vi "Parent.vi"(10 "Label.Text":string, 11 "Parent in":string) -> (3 "Parent out":string)   [LabVIEW 2021, in "Tree.lvlib" / "Tree.lvclass"]
uses:
  Tree.lvclass
  Tree.lvclass/Tree.ctl
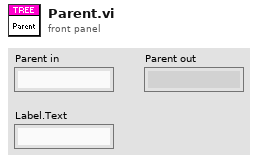
[diagram p1: front panel]
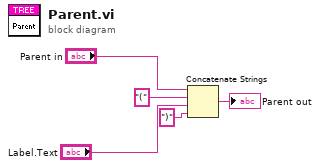
[diagram p0: block diagram]
diagram:
  n1 = Concatenate Strings("Parent in", "(" ("string"), "Label.Text", ")" ("string")) -> (→"Parent out":string)
